vi "main.vi"() -> ()   [LabVIEW 2023] (continued)
2E\t80\tFF\tFF\tFD\r\n      1763  0CF101A7   00000004    8        68\t00\t97\tCC\t00\t16\t39\t72\r\n      1762  1FFFFFFF   00000004    8        00\t00\tFF\tFF\tFF\tFF\tFF\tFF\r\n      1803  0CF102A7   00000004    8        30\t75\tE0\t2E\t80\tFF\tFF\tFD\r\n      1803  0CF101A7   00000004    8        68\t00\t97\tCC\t00\t16\t39\t74\r\n      1802  1FFFFFFF   00000004    8        00\t00\tFF\tFF\tFF\tFF\tFF\tFF\r\n      1793  18F106A7   00000004    8        00\tF7\tFF\tFF\tFF\tFF\tFF\t94\r\n      1792  1FFFFFFF   00000004    8        00\t20\tFF\tFF\tFF\tFF\tFF\tFF\r\n      1783  0CF102A7   00000004    8        30\t75\tE0\t2E\t80\tFF\tFF\tFD\r\n      1783  0CF101A7   00000004    8        68\t00\t97\tCC\t00\t16\t39\t73\r\n      1782  1FFFFFFF   00000004    8        00\t20\tFF\tFF\tFF\tFF\tFF\tFF\r\n      1772  1FFFFFFF   00000004    8        00\t20\tFF\tFF\tFF\tFF\tFF\tFF\r\n      1763  0CF102A7   00000004    8        30\t75\tE0\t2E\t80\tFF\tFF\tFD\r\n      1763  0CF101A7   00000004    8        68\t00\t97\tCC\t00\t16\t39\t72\r\n      1812  1FFFFFFF   00000004    8        00\t20\tFF\tFF\tFF\tFF\tFF\tFF\r\n      1803  0CF102A7   00000004    8        30\t75\tE0\t2E\t80\tFF\tFF\tFD\r\n      1803  0CF101A7   00000004    8        68\t00\t97\tCC\t00\t16\t39\t74\r\n      1802  1FFFFFFF   00000004    8        00\t00\tFF\tFF\tFF\tFF\tFF\tFF\r\n      1793  18F106A7   00000004    8        00\tF7\tFF\tFF\tFF\tFF\tFF\t94\r\n      1792  1FFFFFFF   00000004    8        00\t20\tFF\tFF\tFF\tFF\tFF\tFF\r\n      1783  0CF102A7   00000004    8        30\t75\tE0\t2E\t80\tFF\tFF\tFD\r\n      1783  0CF101A7   00000004    8        68\t00\t97\tCC\t00\t16\t39\t73\r\n      1782  1FFFFFFF   00000004    8        00\t20\tFF\tFF\tFF\tFF\tFF\tFF\r\n      1772  1FFFFFFF   00000004    8        00\t20\tFF\tFF\tFF\tFF\tFF\tFF\r\n      1763  0CF102A7   00000004    8        30\t75\tE0\t2E\t80\tFF\tFF\tFD\r\n      1822  1FFFFFFF   00000004    8        00\t00\tFF\tFF\tFF\tFF\tFF\tFF\r\n      1812  1FFFFFFF   00000004    8        00\t20\tFF\tFF\tFF\tFF\tFF\tFF\r\n      1803  0CF102A7   00000004    8        30\t75\tE0\t2E\t80\tFF\tFF\tFD\r\n      1803  0CF101A7   00000004    8        68\t00\t97\tCC\t00\t16\t39\t74\r\n      1802  1FFFFFFF   00000004    8        00\t00\tFF\tFF\tFF\tFF\tFF\tFF\r\n      1793  18F106A7   00000004    8        00\tF7\tFF\tFF\tFF\tFF\tFF\t94\r\n      1792  1FFFFFFF   00000004    8        00\t20\tFF\tFF\tFF\tFF\tFF\tFF\r\n      1783  0CF102A7   00000004    8        30\t75\tE0\t2E\t80\tFF\tFF\tFD\r\n      1783  0CF101A7   00000004    8        68\t00\t97\tCC\t00\t16\t39\t73\r\n      1782  1FFFFFFF   00000004    8        00\t20\tFF\tFF\tFF\tFF\tFF\tFF\r\n      1772  1FFFFFFF   00000004    8        00\t20\tFF\tFF\tFF\tFF\tFF\tFF\r\n      1823  0CF101A7   00000004    8        68\t00\t97\tCC\t00\t16\t39\t75\r\n      1822  1FFFFFFF   00000004    8        00\t00\tFF\tFF\tFF\tFF\tFF\tFF\r\n      1812  1FFFFFFF   00000004    8        00\t20\tFF\tFF\tFF\tFF\tFF\tFF\r\n      1803  0CF102A7   00000004    8        30\t75\tE0\t2E\t80\tFF\tFF\tFD\r\n      1803  0CF101A7   00000004    8        68\t00\t97\tCC\t00\t16\t39\t74\r\n      1802  1FFFFFFF   00000004    8        00\t00\tFF\tFF\tFF\tFF\tFF\tFF\r\n      1793  18F106A7   00000004    8        00\tF7\tFF\tFF\tFF\tFF\tFF\t94\r\n      1792  1FFFFFFF   00000004    8        00\t20\tFF\tFF\tFF\tFF\tFF\tFF\r\n      1783  0CF102A7   00000004    8        30\t75\tE0\t2E\t80\tFF\tFF\tFD\r\n      1783  0CF101A7   00000004    8        68\t00\t97\tCC\t00\t16\t39\t73\r\n      1782  1FFFFFFF   00000004    8        00\t20\tFF\tFF\tFF\tFF\tFF\tFF\r\n      1823  0CF102A7   00000004    8        30\t75\tE0\t2E\t80\tFF\tFF\tFD\r\n      1823  0CF101A7   00000004    8        68\t00\t97\tCC\t00\t16\t39\t75\r\n      1822  1FFFFFFF   00000004    8        00\t00\tFF\tFF\tFF\tFF\tFF\tFF\r\n      1812  1FFFFFFF   00000004    8        00\t20\tFF\tFF\tFF\tFF\tFF\tFF\r\n      1803  0CF102A7   00000004    8        30\t75\tE0\t2E\t80\tFF\tFF\tFD\r\n      1803  0CF101A7   00000004    8        68\t00\t97\tCC\t00\t16\t39\t74\r\n      1802  1FFFFFFF   00000004    8        00\t00\tFF\tFF\tFF\tFF\tFF\tFF\r\n      1793  18F106A7   00000004    8        00\tF7\tFF\tFF\tFF\tFF\tFF\t94\r\n      1792  1FFFFFFF   00000004    8        00\t20\tFF\tFF\tFF\tFF\tFF\tFF\r\n      1783  0CF102A7   00000004    8        30\t75\tE0\t2E\t80\tFF\tFF\tFD\r\n      1783  0CF101A7   00000004    8        68\t00\t97\tCC\t00\t16\t39\t73\r\n      1832  1FFFFFFF   00000004    8        00\t20\tFF\tFF\tFF\tFF\tFF\tFF\r\n      1823  0CF102A7   00000004    8        30\t75\tE0\t2E\t80\tFF\tFF\tFD\r\n      1823  0CF101A7   00000004    8        68\t00\t97\tCC\t00\t16\t39\t75\r\n      1822  1FFFFFFF   00000004    8        00\t00\tFF\tFF\tFF\tFF\tFF\tFF\r\n      1812  1FFFFFFF   00000004    8        00\t20\tFF\tFF\tFF\tFF\tFF\tFF\r\n      1803  0CF102A7   00000004    8        30\t75\tE0\t2E\t80\tFF\tFF\tFD\r\n      1803  0CF101A7   00000004    8        68\t00\t97\tCC\t00\t16\t39\t74\r\n      1802  1FFFFFFF   00000004    8        00\t00\tFF\tFF\tFF\tFF\tFF\tFF\r\n      1793  18F106A7   00000004    8        00\tF7\tFF\tFF\tFF\tFF\tFF\t94\r\n      1792  1FFFFFFF   00000004    8        00\t20\tFF\tFF\tFF\tFF\tFF\tFF\r\n      1783  0CF102A7   00000004    8        30\t75\tE0\t2E\t80\tFF\tFF\tFD\r\n      1841  18F11FF0   00000004    8        FF\t3F\t90\t68\t88\t1B\t10\tAC\r\n      1832  1FFFFFFF   00000004    8        00\t20\tFF\tFF\tFF\tFF\tFF\tFF\r\n      1823  0CF102A7   00000004    8        30\t75\tE0\t2E\t80\tFF\tFF\tFD\r\n      1823  0CF101A7   00000004    8        68\t00\t97\tCC\t00\t16\t39\t75\r\n      1822  1FFFFFFF   00000004    8        00\t00\tFF\tFF\tFF\tFF\tFF\tFF\r\n      1812  1FFFFFFF   00000004    8        00\t20\tFF\tFF\tFF\tFF\tFF\tFF\r\n      1803  0CF102A7   00000004    8        30\t75\tE0\t2E\t80\tFF\tFF\tFD\r\n      1803  0CF101A7   00000004    8        68\t00\t97\tCC\t00\t16\t39\t74\r\n      1802  1FFFFFFF   00000004    8        00\t00\tFF\tFF\tFF\tFF\tFF\tFF\r\n      1793  18F106A7   00000004    8        00\tF7\tFF\tFF\tFF\tFF\tFF\t94\r\n      1792  1FFFFFFF   00000004    8        00\t20\tFF\tFF\tFF\tFF\tFF\tFF\r\n      1842  18F120F0   00000004    8        2B\t75\t60\tB1\tB0\t01\tFF\tFF\r\n      1841  18F11FF0   00000004    8        FF\t3F\t90\t68\t88\t1B\t10\tAC\r\n      1832  1FFFFFFF   00000004    8        00\t20\tFF\tFF\tFF\tFF\tFF\tFF\r\n      1823  0CF102A7   00000004    8        30\t75\tE0\t2E\t80\tFF\tFF\tFD\r\n      1823  0CF101A7   00000004    8        68\t00\t97\tCC\t00\t16\t39\t75\r\n      1822  1FFFFFFF   00000004    8        00\t00\tFF\tFF\tFF\tFF\tFF\tFF\r\n      1812  1FFFFFFF   00000004    8        00\t20\tFF\tFF\tFF\tFF\tFF\tFF\r\n      1803  0CF102A7   00000004    8        30\t75\tE0\t2E\t80\tFF\tFF\tFD\r\n      1803  0CF101A7   00000004    8        68\t00\t97\tCC\t00\t16\t39\t74\r\n      1802  1FFFFFFF   00000004    8        00\t00\tFF\tFF\tFF\tFF\tFF\tFF\r\n      1793  18F106A7   00000004    8        00\tF7\tFF\tFF\tFF\tFF\tFF\t94\r\n      1843  0CF101A7   00000004    8        68\t00\t97\tCC\t00\t16\t39\t76\r\n      1842  18F120F0   00000004    8        2B\t75\t60\tB1\tB0\t01\tFF\tFF\r\n      1841  18F11FF0   00000004    8        FF\t3F\t90\t68\t88\t1B\t10\tAC\r\n      1832  1FFFFFFF   00000004    8        00\t20\tFF\tFF\tFF\tFF\tFF\tFF\r\n      1823  0CF102A7   00000004    8        30\t75\tE0\t2E\t80\tFF\tFF\tFD\r\n      1823  0CF101A7   00000004    8        68\t00\t97\tCC\t00\t16\t39\t75\r\n      1822  1FFFFFFF   00000004    8        00\t00\tFF\tFF\tFF\tFF\tFF\tFF\r\n      1812  1FFFFFFF   00000004    8        00\t20\tFF\tFF\tFF\tFF\tFF\tFF\r\n      1803  0CF102A7   00000004    8        30\t75\tE0\t2E\t80\tFF\tFF\tFD\r\n      1803  0CF101A7   00000004    8        68\t00\t97\tCC\t00\t16\t39\t74\r\n      1802  1FFFFFFF   00000004    8        00\t00\tFF\tFF\tFF\tFF\tFF\tFF\r\n      1843  0C3C4D4A   00000004    8        BE\tFF\tFF\t7F\t18\tFF\tFF\t4A\r\n      1843  0CF101A7   00000004    8        68\t00\t97\tCC\t00\t16\t39\t76\r\n      1842  18F120F0   00000004    8        2B\t75\t60\tB1\tB0\t01\tFF\tFF\r\n      1841  18F11FF0   00000004    8        FF\t3F\t90\t68\t88\t1B\t10\tAC\r\n      1832  1FFFFFFF   00000004    8        00\t20\tFF\tFF\tFF\tFF\tFF\tFF\r\n      1823  0CF102A7   00000004    8        30\t75\tE0\t2E\t80\tFF\tFF\tFD\r\n      1823  0CF101A7   00000004    8        68\t00\t97\tCC\t00\t16\t39\t75\r\n      1822  1FFFFFFF   00000004    8        00\t00\tFF\tFF\tFF\tFF\tFF\tFF\r\n      1812  1FFFFFFF   00000004    8        00\t20\tFF\tFF\tFF\tFF\tFF\tFF\r\n      1803  0CF102A7   00000004    8        30\t75\tE0\t2E\t80\tFF\tFF\tFD\r\n      1803  0CF101A7   00000004    8        68\t00\t97\tCC\t00\t16\t39\t74\r\n      1844  0CF102A7   00000004    8        30\t75\tE0\t2E\t80\tFF\tFF\tFD\r\n      1843  0C3C4D4A   00000004    8        BE\tFF\tFF\t7F\t18\tFF\tFF\t4A\r\n      1843  0CF101A7   00000004    8        68\t00\t97\tCC\t00\t16\t39\t76\r\n      1842  18F120F0   00000004    8        2B\t75\t60\tB1\tB0\t01\tFF\tFF\r\n      1841  18F11FF0   00000004    8        FF\t3F\t90\t68\t88\t1B\t10\tAC\r\n      1832  1FFFFFFF   00000004    8        00\t20\tFF\tFF\tFF\tFF\tFF\tFF\r\n      1823  0CF102A7   00000004    8        30\t75\tE0\t2E\t80\tFF\tFF\tFD\r\n      1823  0CF101A7   00000004    8        68\t00\t97\tCC\t00\t16\t39\t75\r\n      1822  1FFFFFFF   00000004    8        00\t00\tFF\tFF\tFF\tFF\tFF\tFF\r\n      1812  1FFFFFFF   00000004    8        00\t20\tFF\tFF\tFF\tFF\tFF\tFF\r\n      1803  0CF102A7   00000004    8        30\t75\tE0\t2E\t80\tFF\tFF\tFD\r\n      1844  0CF103A7   00000004    8        17\t1F\t08\t60\tB1\t1F\t08\t4A\r\n      1844  0CF102A7   00000004    8        30\t75\tE0\t2E\t80\tFF\tFF\tFD\r\n      1843  0C3C4D4A   00000004    8        BE\tFF\tFF\t7F\t18\tFF\tFF\t4A\r\n      1843  0CF101A7   00000004    8        68\t00\t97\tCC\t00\t16\t39\t76\r\n      1842  18F120F0   00000004    8        2B\t75\t60\tB1\tB0\t01\tFF\tFF\r\n      1841  18F11FF0   00000004    8        FF\t3F\t90\t68\t88\t1B\t10\tAC\r\n      1832  1FFFFFFF   00000004    8        00\t20\tFF\tFF\tFF\tFF\tFF\tFF\r\n      1823  0CF102A7   00000004    8        30\t75\tE0\t2E\t80\tFF\tFF\tFD\r\n      1823  0CF101A7   00000004    8        68\t00\t97\tCC\t00\t16\t39\t75\r\n      1822  1FFFFFFF   00000004    8        00\t00\tFF\tFF\tFF\tFF\tFF\tFF\r\n      1812  1FFFFFFF   00000004    8        00\t20\tFF\tFF\tFF\tFF\tFF\tFF\r\n      1845  0CF104A7   00000004    8        F0\t60\t22\tFC\tFF\tFF\tFF\t4A\r\n      1844  0CF103A7   00000004    8        17\t1F\t08\t60\tB1\t1F\t08\t4A\r\n      1844  0CF102A7   00000004    8        30\t75\tE0\t2E\t80\tFF\tFF\tFD\r\n      1843  0C3C4D4A   00000004    8        BE\tFF\tFF\t7F\t18\tFF\tFF\t4A\r\n      1843  0CF101A7   00000004    8        68\t00\t97\tCC\t00\t16\t39\t76\r\n      1842  18F120F0   00000004    8        2B\t75\t60\tB1\tB0\t01\tFF\tFF\r\n      1841  18F11FF0   00000004    8        FF\t3F\t90\t68\t88\t1B\t10\tAC\r\n      1832  1FFFFFFF   00000004    8        00\t20\tFF\tFF\tFF\tFF\tFF\tFF\r\n      1823  0CF102A7   00000004    8        30\t75\tE0\t2E\t80\tFF\tFF\tFD\r\n      1823  0CF101A7   00000004    8        68\t00\t97\tCC\t00\t16\t39\t75\r\n      1822  1FFFFFFF   00000004    8        00\t00\tFF\tFF\tFF\tFF\tFF\tFF\r\n      1845  18F106A7   00000004    8        00\tF7\tFF\tFF\tFF\tFF\tFF\t95\r\n      1845  0CF104A7   00000004    8        F0\t60\t22\tFC\tFF\tFF\tFF\t4A\r\n      1844  0CF103A7   00000004    8        17\t1F\t08\t60\tB1\t1F\t08\t4A\r\n      1844  0CF102A7   00000004    8        30\t75\tE0\t2E\t80\tFF\tFF\tFD\r\n      1843  0C3C4D4A   00000004    8        BE\tFF\tFF\t7F\t18\tFF\tFF\t4A\r\n      1843  0CF101A7   00000004    8        68\t00\t97\tCC\t00\t16\t39\t76\r\n      1842  18F120F0   00000004    8        2B\t75\t60\tB1\tB0\t01\tFF\tFF\r\n      1841  18F11FF0   00000004    8        FF\t3F\t90\t68\t88\t1B\t10\tAC\r\n      1832  1FFFFFFF   00000004    8        00\t20\tFF\tFF\tFF\tFF\tFF\tFF\r\n      1823  0CF102A7   00000004    8        30\t75\tE0\t2E\t80\tFF\tFF\tFD\r\n      1823  0CF101A7   00000004    8        68\t00\t97\tCC\t00\t16\t39\t75\r\n      1846  18F121F0   00000004    8        09\t18\t00\t00\tFF\tFF\tB0\t01\r\n      1845  18F106A7   00000004    8        00\tF7\tFF\tFF\tFF\tFF\tFF\t95\r\n      1845  0CF104A7   00000004    8        F0\t60\t22\tFC\tFF\tFF\tFF\t4A\r\n      1844  0CF103A7   00000004    8        17\t1F\t08\t60\tB1\t1F\t08\t4A\r\n      1844  0CF102A7   00000004    8        30\t75\tE0\t2E\t80\tFF\tFF\tFD\r\n      1843  0C3C4D4A   00000004    8        BE\tFF\tFF\t7F\t18\tFF\tFF\t4A\r\n      1843  0CF101A7   00000004    8        68\t00\t97\tCC\t00\t16\t39\t76\r\n      1842  18F120F0   00000004    8        2B\t75\t60\tB1\tB0\t01\tFF\tFF\r\n      1841  18F11FF0   00000004    8        FF\t3F\t90\t68\t88\t1B\t10\tAC\r\n      1832  1FFFFFFF   00000004    8        00\t20\tFF\tFF\tFF\tFF\tFF\tFF\r\n      1823  0CF102A7   00000004    8        30\t75\tE0\t2E\t80\tFF\tFF\tFD\r\n      1847  1FFFFFFF   00000004    8        00\t00\tFF\tFF\tFF\tFF\tFF\tFF\r\n      1846  18F121F0   00000004    8        09\t18\t00\t00\tFF\tFF\tB0\t01\r\n      1845  18F106A7   00000004    8        00\tF7\tFF\tFF\tFF\tFF\tFF\t95\r\n      1845  0CF104A7   00000004    8        F0\t60\t22\tFC\tFF\tFF\tFF\t4A\r\n      1844  0CF103A7   00000004    8        17\t1F\t08\t60\tB1\t1F\t08\t4A\r\n      1844  0CF102A7   00000004    8        30\t75\tE0\t2E\t80\tFF\tFF\tFD\r\n      1843  0C3C4D4A   00000004    8        BE\tFF\tFF\t7F\t18\tFF\tFF\t4A\r\n      1843  0CF101A7   00000004    8        68\t00\t97\tCC\t00\t16\t39\t76\r\n      1842  18F120F0   00000004    8        2B\t75\t60\tB1\tB0\t01\tFF\tFF\r\n      1841  18F11FF0   00000004    8        FF\t3F\t90\t68\t88\t1B\t10\tAC\r\n      1832  1FFFFFFF   00000004    8        00\t20\tFF\tFF\tFF\tFF\tFF\tFF\r\n      1852  1FFFFFFF   00000004    8        00\t20\tFF\tFF\tFF\tFF\tFF\tFF\r\n      1847  1FFFFFFF   00000004    8        00\t00\tFF\tFF\tFF\tFF\tFF\tFF\r\n      1846  18F121F0   00000004    8        09\t18\t00\t00\tFF\tFF\tB0\t01\r\n      1845  18F106A7   00000004    8        00\tF7\tFF\tFF\tFF\tFF\tFF\t95\r\n      1845  0CF104A7   00000004    8        F0\t60\t22\tFC\tFF\tFF\tFF\t4A\r\n      1844  0CF103A7   00000004    8        17\t1F\t08\t60\tB1\t1F\t08\t4A\r\n      1844  0CF102A7   00000004    8        30\t75\tE0\t2E\t80\tFF\tFF\tFD\r\n      1843  0C3C4D4A   00000004    8        BE\tFF\tFF\t7F\t18\tFF\tFF\t4A\r\n      1843  0CF101A7   00000004    8        68\t00\t97\tCC\t00\t16\t39\t76\r\n      1842  18F120F0   00000004    8        2B\t75\t60\tB1\tB0\t01\tFF\tFF\r\n      1841  18F11FF0   00000004    8        FF\t3F\t90\t68\t88\t1B\t10\tAC\r\n      1862  1FFFFFFF   00000004    8        00\t20\tFF\tFF\tFF\tFF\tFF\tFF\r\n      1852  1FFFFFFF   00000004    8        00\t20\tFF\tFF\tFF\tFF\tFF\tFF\r\n      1847  1FFFFFFF   00000004    8        00\t00\tFF\tFF\tFF\tFF\tFF\tFF\r\n      1846  18F121F0   00000004    8        09\t18\t00\t00\tFF\tFF\tB0\t01\r\n      1845  18F106A7   00000004    8        00\tF7\tFF\tFF\tFF\tFF\tFF\t95\r\n      1845  0CF104A7   00000004    8        F0\t60\t22\tFC\tFF\tFF\tFF\t4A\r\n      1844  0CF103A7   00000004    8        17\t1F\t08\t60\tB1\t1F\t08\t4A\r\n      1844  0CF102A7   00000004    8        30\t75\tE0\t2E\t80\tFF\tFF\tFD\r\n      1843  0C3C4D4A   00000004    8        BE\tFF\tFF\t7F\t18\tFF\tFF\t4A\r\n      1843  0CF101A7   00000004    8        68\t00\t97\tCC\t00\t16\t39\t76\r\n      1842  18F120F0   00000004    8        2B\t75\t60\tB1\tB0\t01\tFF\tFF\r\n      1863  0CF101A7   00000004    8        68\t00\t97\tCC\t00\t16\t39\t77\r\n      1862  1FFFFFFF   00000004    8        00\t20\tFF\tFF\tFF\tFF\tFF\tFF\r\n      1852  1FFFFFFF   00000004    8        00\t20\tFF\tFF\tFF\tFF\tFF\tFF\r\n      1847  1FFFFFFF   00000004    8        00\t00\tFF\tFF\tFF\tFF\tFF\tFF\r\n      1846  18F121F0   00000004    8        09\t18\t00\t00\tFF\tFF\tB0\t01\r\n      1845  18F106A7   00000004    8        00\tF7\tFF\tFF\tFF\tFF\tFF\t95\r\n      1845  0CF104A7   00000004    8        F0\t60\t22\tFC\tFF\tFF\tFF\t4A\r\n      1844  0CF103A7   00000004    8        17\t1F\t08\t60\tB1\t1F\t08\t4A\r\n      1844  0CF102A7   00000004    8        30\t75\tE0\t2E\t80\tFF\tFF\tFD\r\n      1843  0C3C4D4A   00000004    8        BE\tFF\tFF\t7F\t18\tFF\tFF\t4A\r\n      1843  0CF101A7   00000004    8        68\t00\t97\tCC\t00\t16\t39\t76\r\n      1863  0CF102A7   00000004    8        30\t75\tE0\t2E\t80\tFF\tFF\tFD\r\n      1863  0CF101A7   00000004    8        68\t00\t97\tCC\t00\t16\t39\t77\r\n      1862  1FFFFFFF   00000004    8        00\t20\tFF\tFF\tFF\tFF\tFF\tFF\r\n      1852  1FFFFFFF   00000004    8        00\t20\tFF\tFF\tFF\tFF\tFF\tFF\r\n      1847  1FFFFFFF   00000004    8        00\t00\tFF\tFF\tFF\tFF\tFF\tFF\r\n      1846  18F121F0   00000004    8        09\t18\t00\t00\tFF\tFF\tB0\t01\r\n      1845  18F106A7   00000004    8        00\tF7\tFF\tFF\tFF\tFF\tFF\t95\r\n      1845  0CF104A7   00000004    8        F0\t60\t22\tFC\tFF\tFF\tFF\t4A\r\n      1844  0CF103A7   00000004    8        17\t1F\t08\t60\tB1\t1F\t08\t4A\r\n      1844  0CF102A7   00000004    8        30\t75\tE0\t2E\t80\tFF\tFF\tFD\r\n      1843  0C3C4D4A   00000004    8        BE\tFF\tFF\t7F\t18\tFF\tFF\t4A\r\n      1872  1FFFFFFF   00000004    8        00\t20\tFF\tFF\tFF\tFF\tFF\tFF\r\n      1863  0CF102A7   00000004    8        30\t75\tE0\t2E\t80\tFF\tFF\tFD\r\n      1863  0CF101A7   00000004    8        68\t00\t97\tCC\t00\t16\t39\t77\r\n      1862  1FFFFFFF   00000004    8        00\t20\tFF\tFF\tFF\tFF\tFF\tFF\r\n      1852  1FFFFFFF   00000004    8        00\t20\tFF\tFF\tFF\tFF\tFF\tFF\r\n      1847  1FFFFFFF   00000004    8        00\t00\tFF\tFF\tFF\tFF\tFF\tFF\r\n      1846  18F121F0   00000004    8        09\t18\t00\t00\tFF\tFF\tB0\t01\r\n      1845  18F106A7   00000004    8        00\tF7\tFF\tFF\tFF\tFF\tFF\t95\r\n      1845  0CF104A7   00000004    8        F0\t60\t22\tFC\tFF\tFF\tFF\t4A\r\n      1844  0CF103A7   00000004    8        17\t1F\t08\t60\tB1\t1F\t08\t4A\r\n      1844  0CF102A7   00000004    8        30\t75\tE0\t2E\t80\tFF\tFF\tFD\r\n      1882  1FFFFFFF   00000004    8        00\t20\tFF\tFF\tFF\tFF\tFF\tFF\r\n      1872  1FFFFFFF   00000004    8        00\t20\tFF\tFF\tFF\tFF\tFF\tFF\r\n      1863  0CF102A7   00000004    8        30\t75\tE0\t2E\t80\tFF\tFF\tFD\r\n      1863  0CF101A7   00000004    8        68\t00\t97\tCC\t00\t16\t39\t77\r\n      1862  1FFFFFFF   00000004    8        00\t20\tFF\tFF\tFF\tFF\tFF\tFF\r\n      1852  1FFFFFFF   00000004    8        00\t20\tFF\tFF\tFF\tFF\tFF\tFF\r\n      1847  1FFFFFFF   00000004    8        00\t00\tFF\tFF\tFF\tFF\tFF\tFF\r\n      1846  18F121F0   00000004    8        09\t18\t00\t00\tFF\tFF\tB0\t01\r\n      1845  18F106A7   00000004    8        00\tF7\tFF\tFF\tFF\tFF\tFF\t95\r\n      1845  0CF104A7   00000004    8        F0\t60\t22\tFC\tFF\tFF\tFF\t4A\r\n      1844  0CF103A7   00000004    8        17\t1F\t08\t60\tB1\t1F\t08\t4A\r\n      1883  0CF101A7   00000004    8        68\t00\t97\tCC\t00\t16\t39\t78\r\n      1882  1FFFFFFF   00000004    8        00\t20\tFF\tFF\tFF\tFF\tFF\tFF\r\n      1872  1FFFFFFF   00000004    8        00\t20\tFF\tFF\tFF\tFF\tFF\tFF\r\n      1863  0CF102A7   00000004    8        30\t75\tE0\t2E\t80\tFF\tFF\tFD\r\n      1863  0CF101A7   00000004    8        68\t00\t97\tCC\t00\t16\t39\t77\r\n      1862  1FFFFFFF   00000004    8        00\t20\tFF\tFF\tFF\tFF\tFF\tFF\r\n      1852  1FFFFFFF   00000004    8        00\t20\tFF\tFF\tFF\tFF\tFF\tFF\r\n      1847  1FFFFFFF   00000004    8        00\t00\tFF\tFF\tFF\tFF\tFF\tFF\r\n      1846  18F121F0   00000004    8        09\t18\t00\t00\tFF\tFF\tB0\t01\r\n      1845  18F106A7   00000004    8        00\tF7\tFF\tFF\tFF\tFF\tFF\t95\r\n      1845  0CF104A7   00000004    8        F0\t60\t22\tFC\tFF\tFF\tFF\t4A\r\n      1883  0CF102A7   00000004    8        30\t75\tE0\t2E\t80\tFF\tFF\tFD\r\n      1883  0CF101A7   00000004    8        68\t00\t97\tCC\t00\t16\t39\t78\r\n      1882  1FFFFFFF   00000004    8        00\t20\tFF\tFF\tFF\tFF\tFF\tFF\r\n      1872  1FFFFFFF   00000004    8        00\t20\tFF\tFF\tFF\tFF\tFF\tFF\r\n      1863  0CF102A7   00000004    8        30\t75\tE0\t2E\t80\tFF\tFF\tFD\r\n      1863  0CF101A7   00000004    8        68\t00\t97\tCC\t00\t16\t39\t77\r\n      1862  1FFFFFFF   00000004    8        00\t20\tFF\tFF\tFF\tFF\tFF\tFF\r\n      1852  1FFFFFFF   00000004    8        00\t20\tFF\tFF\tFF\tFF\tFF\tFF\r\n      1847  1FFFFFFF   00000004    8        00\t00\tFF\tFF\tFF\tFF\tFF\tFF\r\n      1846  18F121F0   00000004    8        09\t18\t00\t00\tFF\tFF\tB0\t01\r\n      1845  18F106A7   00000004    8        00\tF7\tFF\tFF\tFF\tFF\tFF\t95\r\n      1892  1FFFFFFF   00000004    8        00\t00\tFF\tFF\tFF\tFF\tFF\tFF\r\n      1883  0CF102A7   00000004    8        30\t75\tE0\t2E\t80\tFF\tFF\tFD\r\n      1883  0CF101A7   00000004    8        68\t00\t97\tCC\t00\t16\t39\t78\r\n      1882  1FFFFFFF   00000004    8        00\t20\tFF\tFF\tFF\tFF\tFF\tFF\r\n      1872  1FFFFFFF   00000004    8        00\t20\tFF\tFF\tFF\tFF\tFF\tFF\r\n      1863  0CF102A7   00000004    8        30\t75\tE0\t2E\t80\tFF\tFF\tFD\r\n      1863  0CF101A7   00000004    8        68\t00\t97\tCC\t00\t16\t39\t77\r\n      1862  1FFFFFFF   00000004    8        00\t20\tFF\tFF\tFF\tFF\tFF\tFF\r\n      1852  1FFFFFFF   00000004    8        00\t20\tFF\tFF\tFF\tFF\tFF\tFF\r\n      1847  1FFFFFFF   00000004    8        00\t00\tFF\tFF\tFF\tFF\tFF\tFF\r\n      1846  18F121F0   00000004    8        09\t18\t00\t00\tFF\tFF\tB0\t01\r\n      1893  18F106A7   00000004    8        00\tF7\tFF\tFF\tFF\tFF\tFF\t96\r\n      1892  1FFFFFFF   00000004    8        00\t00\tFF\tFF\tFF\tFF\tFF\tFF\r\n      1883  0CF102A7   00000004    8        30\t75\tE0\t2E\t80\tFF\tFF\tFD\r\n      1883  0CF101A7   00000004    8        68\t00\t97\tCC\t00\t16\t39\t78\r\n      1882  1FFFFFFF   00000004    8        00\t20\tFF\tFF\tFF\tFF\tFF\tFF\r\n      1872  1FFFFFFF   00000004    8        00\t20\tFF\tFF\tFF\tFF\tFF\tFF\r\n      1863  0CF102A7   00000004    8        30\t75\tE0\t2E\t80\tFF\tFF\tFD\r\n      1863  0CF101A7   00000004    8        68\t00\t97\tCC\t00\t16\t39\t77\r\n      1862  1FFFFFFF   00000004    8        00\t20\tFF\tFF\tFF\tFF\tFF\tFF\r\n      1852  1FFFFFFF   00000004    8        00\t20\tFF\tFF\tFF\tFF\tFF\tFF\r\n      1847  1FFFFFFF   00000004    8        00\t00\tFF\tFF\tFF\tFF\tFF\tFF\r\n      1902  1FFFFFFF   00000004    8        00\t20\tFF\tFF\tFF\tFF\tFF\tFF\r\n      1893  18F106A7   00000004    8        00\tF7\tFF\tFF\tFF\tFF\tFF\t96\r\n      1892  1FFFFFFF   00000004    8        00\t00\tFF\tFF\tFF\tFF\tFF\tFF\r\n      1883  0CF102A7   00000004    8        30\t75\tE0\t2E\t80\tFF\tFF\tFD\r\n      1883  0CF101A7   00000004    8        68\t00\t97\tCC\t00\t16\t39\t78\r\n      1882  1FFFFFFF   00000004    8        00\t20\tFF\tFF\tFF\tFF\tFF\tFF\r\n      1872  1FFFFFFF   00000004    8        00\t20\tFF\tFF\tFF\tFF\tFF\tFF\r\n      1863  0CF102A7   00000004    8        30\t75\tE0\t2E\t80\tFF\tFF\tFD\r\n      1863  0CF101A7   00000004    8        68\t00\t97\tCC\t00\t16\t39\t77\r\n      1862  1FFFFFFF   00000004    8        00\t20\tFF\tFF\tFF\tFF\tFF\tFF\r\n      1852  1FFFFFFF   00000004    8        00\t20\tFF\tFF\tFF\tFF\tFF\tFF\r\n      1903  0CF101A7   00000004    8        68\t00\t97\tCC\t00\t16\t39\t79\r\n      1902  1FFFFFFF   00000004    8        00\t20\tFF\tFF\tFF\tFF\tFF\tFF\r\n      1893  18F106A7   00000004    8        00\tF7\tFF\tFF\tFF\tFF\tFF\t96\r\n      1892  1FFFFFFF   00000004    8        00\t00\tFF\tFF\tFF\tFF\tFF\tFF\r\n      1883  0CF102A7   00000004    8        30\t75\tE0\t2E\t80\tFF\tFF\tFD\r\n      1883  0CF101A7   00000004    8        68\t00\t97\tCC\t00\t16\t39\t78\r\n      1882  1FFFFFFF   00000004    8        00\t20\tFF\tFF\tFF\tFF\tFF\tFF\r\n      1872  1FFFFFFF   00000004    8        00\t20\tFF\tFF\tFF\tFF\tFF\tFF\r\n      1863  0CF102A7   00000004    8        30\t75\tE0\t2E\t80\tFF\tFF\tFD\r\n      1863  0CF101A7   00000004    8        68\t00\t97\tCC\t00\t16\t39\t77\r\n      1862  1FFFFFFF   00000004    8        00\t20\tFF\tFF\tFF\tFF\tFF\tFF\r\n      1903  0CF102A7   00000004    8        30\t75\tE0\t2E\t80\tFF\tFF\tFD\r\n      1903  0CF101A7   00000004    8        68\t00\t97\tCC\t00\t16\t39\t79\r\n      1902  1FFFFFFF   00000004    8        00\t20\tFF\tFF\tFF\tFF\tFF\tFF\r\n      1893  18F106A7   00000004    8        00\tF7\tFF\tFF\tFF\tFF\tFF\t96\r\n      1892  1FFFFFFF   00000004    8        00\t00\tFF\tFF\tFF\tFF\tFF\tFF\r\n      1883  0CF102A7   00000004    8        30\t75\tE0\t2E\t80\tFF\tFF\tFD\r\n      1883  0CF101A7   00000004    8        68\t00\t97\tCC\t00\t16\t39\t78\r\n      1882  1FFFFFFF   00000004    8        00\t20\tFF\tFF\tFF\tFF\tFF\tFF\r\n      1872  1FFFFFFF   00000004    8        00\t20\tFF\tFF\tFF\tFF\tFF\tFF\r\n      1863  0CF102A7   00000004    8        30\t75\tE0\t2E\t80\tFF\tFF\tFD\r\n      1863  0CF101A7   00000004    8        68\t00\t97\tCC\t00\t16\t39\t77\r\n      1912  1FFFFFFF   00000004    8        00\t00\tFF\tFF\tFF\tFF\tFF\tFF\r\n      1903  0CF102A7   00000004    8        30\t75\tE0\t2E\t80\tFF\tFF\tFD\r\n      1903  0CF101A7   00000004    8        68\t00\t97\tCC\t00\t16\t39\t79\r\n      1902  1FFFFFFF   00000004    8        00\t20\tFF\tFF\tFF\tFF\tFF\tFF\r\n      1893  18F106A7   00000004    8        00\tF7\tFF\tFF\tFF\tFF\tFF\t96\r\n      1892  1FFFFFFF   00000004    8        00\t00\tFF\tFF\tFF\tFF\tFF\tFF\r\n      1883  0CF102A7   00000004    8        30\t75\tE0\t2E\t80\tFF\tFF\tFD\r\n      1883  0CF101A7   00000004    8        68\t00\t97\tCC\t00\t16\t39\t78\r\n      1882  1FFFFFFF   00000004    8        00\t20\tFF\tFF\tFF\tFF\tFF\tFF\r\n      1872  1FFFFFFF   00000004    8        00\t20\tFF\tFF\tFF\tFF\tFF\tFF\r\n      1863  0CF102A7   00000004    8        30\t75\tE0\t2E\t80\tFF\tFF\tFD\r\n      1922  1FFFFFFF   00000004    8        00\t20\tFF\tFF\tFF\tFF\tFF\tFF\r\n      1912  1FFFFFFF   00000004    8        00\t00\tFF\tFF\tFF\tFF\tFF\tFF\r\n      1903  0CF102A7   00000004    8        30\t75\tE0\t2E\t80\tFF\tFF\tFD\r\n      1903  0CF101A7   00000004    8        68\t00\t97\tCC\t00\t16\t39\t79\r\n      1902  1FFFFFFF   00000004    8        00\t20\tFF\tFF\tFF\tFF\tFF\tFF\r\n      1893  18F106A7   00000004    8        00\tF7\tFF\tFF\tFF\tFF\tFF\t96\r\n      1892  1FFFFFFF   00000004    8        00\t00\tFF\tFF\tFF\tFF\tFF\tFF\r\n      1883  0CF102A7   00000004    8        30\t75\tE0\t2E\t80\tFF\tFF\tFD\r\n      1883  0CF101A7   00000004    8        68\t00\t97\tCC\t00\t16\t39\t78\r\n      1882  1FFFFFFF   00000004    8        00\t20\tFF\tFF\tFF\tFF\tFF\tFF\r\n      1872  1FFFFFFF   00000004    8        00\t20\tFF\tFF\tFF\tFF\tFF\tFF\r\n      1923  0CF101A7   00000004    8        68\t00\t97\tCC\t00\t16\t39\t7A\r\n      1922  1FFFFFFF   00000004    8        00\t20\tFF\tFF\tFF\tFF\tFF\tFF\r\n      1912  1FFFFFFF   00000004    8        00\t00\tFF\tFF\tFF\tFF\tFF\tFF\r\n      1903  0CF102A7   00000004    8        30\t75\tE0\t2E\t80\tFF\tFF\tFD\r\n      1903  0CF101A7   00000004    8        68\t00\t97\tCC\t00\t16\t39\t79\r\n      1902  1FFFFFFF   00000004    8        00\t20\tFF\tFF\tFF\tFF\tFF\tFF\r\n      1893  18F106A7   00000004    8        00\tF7\tFF\tFF\tFF\tFF\tFF\t96\r\n      1892  1FFFFFFF   00000004    8        00\t00\tFF\tFF\tFF\tFF\tFF\tFF\r\n      1883  0CF102A7   00000004    8        30\t75\tE0\t2E\t80\tFF\tFF\tFD\r\n      1883  0CF101A7   00000004    8        68\t00\t97\tCC\t00\t16\t39\t78\r\n      1882  1FFFFFFF   00000004    8        00\t20\tFF\tFF\tFF\tFF\tFF\tFF\r\n      1923  0CF102A7   00000004    8        30\t75\tE0\t2E\t80\tFF\tFF\tFD\r\n      1923  0CF101A7   00000004    8        68\t00\t97\tCC\t00\t16\t39\t7A\r\n      1922  1FFFFFFF   00000004    8        00\t20\tFF\tFF\tFF\tFF\tFF\tFF\r\n      1912  1FFFFFFF   00000004    8        00\t00\tFF\tFF\tFF\tFF\tFF\tFF\r\n      1903  0CF102A7   00000004    8        30\t75\tE0\t2E\t80\tFF\tFF\tFD\r\n      1903  0CF101A7   00000004    8        68\t00\t97\tCC\t00\t16\t39\t79\r\n      1902  1FFFFFFF   00000004    8        00\t20\tFF\tFF\tFF\tFF\tFF\tFF\r\n      1893  18F106A7   00000004    8        00\tF7\tFF\tFF\tFF\tFF\tFF\t96\r\n      1892  1FFFFFFF   00000004    8        00\t00\tFF\tFF\tFF\tFF\tFF\tFF\r\n      1883  0CF102A7   00000004    8        30\t75\tE0\t2E\t80\tFF\tFF\tFD\r\n      1883  0CF101A7   00000004    8        68\t00\t97\tCC\t00\t16\t39\t78\r\n      1932  1FFFFFFF   00000004    8        00\t20\tFF\tFF\tFF\tFF\tFF\tFF\r\n      1923  0CF102A7   00000004    8        30\t75\tE0\t2E\t80\tFF\tFF\tFD\r\n      1923  0CF101A7   00000004    8        68\t00\t97\tCC\t00\t16\t39\t7A\r\n      1922  1FFFFFFF   00000004    8        00\t20\tFF\tFF\tFF\tFF\tFF\tFF\r\n      1912  1FFFFFFF   00000004    8        00\t00\tFF\tFF\tFF\tFF\tFF\tFF\r\n      1903  0CF102A7   00000004    8        30\t75\tE0\t2E\t80\tFF\tFF\tFD\r\n      1903  0CF101A7   00000004    8        68\t00\t97\tCC\t00\t16\t39\t79\r\n      1902  1FFFFFFF   00000004    8        00\t20\tFF\tFF\tFF\tFF\tFF\tFF\r\n      1893  18F106A7   00000004    8        00\tF7\tFF\tFF\tFF\tFF\tFF\t96\r\n      1892  1FFFFFFF   00000004    8        00\t00\tFF\tFF\tFF\tFF\tFF\tFF\r\n      1883  0CF102A7   00000004    8        30\t75\tE0\t2E\t80\tFF\tFF\tFD\r\n      1941  18F11FF0   00000004    8        FF\t3F\t90\t68\t88\t1B\t10\tBC\r\n      1932  1FFFFFFF   00000004    8        00\t20\tFF\tFF\tFF\tFF\tFF\tFF\r\n      1923  0CF102A7   00000004    8        30\t75\tE0\t2E\t80\tFF\tFF\tFD\r\n      1923  0CF101A7   00000004    8        68\t00\t97\tCC\t00\t16\t39\t7A\r\n      1922  1FFFFFFF   00000004    8        00\t20\tFF\tFF\tFF\tFF\tFF\tFF\r\n      1912  1FFFFFFF   00000004    8        00\t00\tFF\tFF\tFF\tFF\tFF\tFF\r\n      1903  0CF102A7   00000004    8        30\t75\tE0\t2E\t80\tFF\tFF\tFD\r\n      1903  0CF101A7   00000004    8        68\t00\t97\tCC\t00\t16\t39\t79\r\n      1902  1FFFFFFF   00000004    8        00\t20\tFF\tFF\tFF\tFF\tFF\tFF\r\n      1893  18F106A7   00000004    8        00\tF7\tFF\tFF\tFF\tFF\tFF\t96\r\n      1892  1FFFFFFF   00000004    8        00\t00\tFF\tFF\tFF\tFF\tFF\tFF\r\n      1942  18F120F0   00000004    8        2B\t75\t60\tB1\tB0\t01\tFF\tFF\r\n      1941  18F11FF0   00000004    8        FF\t3F\t90\t68\t88\t1B\t10\tBC\r\n      1932  1FFFFFFF   00000004    8        00\t20\tFF\tFF\tFF\tFF\tFF\tFF\r\n      1923  0CF102A7   00000004    8        30\t75\tE0\t2E\t80\tFF\tFF\tFD\r\n      1923  0CF101A7   00000004    8        68\t00\t97\tCC\t00\t16\t39\t7A\r\n      1922  1FFFFFFF   00000004    8        00\t20\tFF\tFF\tFF\tFF\tFF\tFF\r\n      1912  1FFFFFFF   00000004    8        00\t00\tFF\tFF\tFF\tFF\tFF\tFF\r\n      1903  0CF102A7   00000004    8        30\t75\tE0\t2E\t80\tFF\tFF\tFD\r\n      1903  0CF101A7   00000004    8        68\t00\t97\tCC\t00\t16\t39\t79\r\n      1902  1FFFFFFF   00000004    8        00\t20\tFF\tFF\tFF\tFF\tFF\tFF\r\n      1893  18F106A7   00000004    8        00\tF7\tFF\tFF\tFF\tFF\tFF\t96\r\n      1943  0CF101A7   00000004    8        68\t00\t97\tCC\t00\t16\t39\t7B\r\n      1942  18F120F0   00000004    8        2B\t75\t60\tB1\tB0\t01\tFF\tFF\r\n      1941  18F11FF0   00000004    8        FF\t3F\t90\t68\t88\t1B\t10\tBC\r\n      1932  1FFFFFFF   00000004    8        00\t20\tFF\tFF\tFF\tFF\tFF\tFF\r\n      1923  0CF102A7   00000004    8        30\t75\tE0\t2E\t80\tFF\tFF\tFD\r\n      1923  0CF101A7   00000004    8        68\t00\t97\tCC\t00\t16\t39\t7A\r\n      1922  1FFFFFFF   00000004    8        00\t20\tFF\tFF\tFF\tFF\tFF\tFF\r\n      1912  1FFFFFFF   00000004    8        00\t00\tFF\tFF\tFF\tFF\tFF\tFF\r\n      1903  0CF102A7   00000004    8        30\t75\tE0\t2E\t80\tFF\tFF\tFD\r\n      1903  0CF101A7   00000004    8        68\t00\t97\tCC\t00\t16\t39\t79\r\n      1902  1FFFFFFF   00000004    8        00\t20\tFF\tFF\tFF\tFF\tFF\tFF\r\n      1943  0C3C4D4A   00000004    8        BE\tFF\tFF\t7F\t18\tFF\tFF\t4B\r\n      1943  0CF101A7   00000004    8        68\t00\t97\tCC\t00\t16\t39\t7B\r\n      1942  18F120F0   00000004    8        2B\t75\t60\tB1\tB0\t01\tFF\tFF\r\n      1941  18F11FF0   00000004    8        FF\t3F\t90\t68\t88\t1B\t10\tBC\r\n      1932  1FFFFFFF   00000004    8        00\t20\tFF\tFF\tFF\tFF\tFF\tFF\r\n      1923  0CF102A7   00000004    8        30\t75\tE0\t2E\t80\tFF\tFF\tFD\r\n      1923  0CF101A7   00000004    8        68\t00\t97\tCC\t00\t16\t39\t7A\r\n      1922  1FFFFFFF   00000004    8        00\t20\tFF\tFF\tFF\tFF\tFF\tFF\r\n      1912  1FFFFFFF   00000004    8        00\t00\tFF\tFF\tFF\tFF\tFF\tFF\r\n      1903  0CF102A7   00000004    8        30\t75\tE0\t2E\t80\tFF\tFF\tFD\r\n      1903  0CF101A7   00000004    8        68\t00\t97\tCC\t00\t16\t39\t79\r\n      1944  0CF102A7   00000004    8        30\t75\tE0\t2E\t80\tFF\tFF\tFD\r\n      1943  0C3C4D4A   00000004    8        BE\tFF\tFF\t7F\t18\tFF\tFF\t4B\r\n      1943  0CF101A7   00000004    8        68\t00\t97\tCC\t00\t16\t39\t7B\r\n      1942  18F120F0   00000004    8        2B\t75\t60\tB1\tB0\t01\tFF\tFF\r\n      1941  18F11FF0   00000004    8        FF\t3F\t90\t68\t88\t1B\t10\tBC\r\n      1932  1FFFFFFF   00000004    8        00\t20\tFF\tFF\tFF\tFF\tFF\tFF\r\n      1923  0CF102A7   00000004    8        30\t75\tE0\t2E\t80\tFF\tFF\tFD\r\n      1923  0CF101A7   00000004    8        68\t00\t97\tCC\t00\t16\t39\t7A\r\n      1922  1FFFFFFF   00000004    8        00\t20\tFF\tFF\tFF\tFF\tFF\tFF\r\n      1912  1FFFFFFF   00000004    8        00\t00\tFF\tFF\tFF\tFF\tFF\tFF\r\n      1903  0CF102A7   00000004    8        30\t75\tE0\t2E\t80\tFF\tFF\tFD\r\n      1944  0CF103A7   00000004    8        17\t1F\t08\t60\tB1\t1F\t08\t4B\r\n      1944  0CF102A7   00000004    8        30\t75\tE0\t2E\t80\tFF\tFF\tFD\r\n      1943  0C3C4D4A   00000004    8        BE\tFF\tFF\t7F\t18\tFF\tFF\t4B\r\n      1943  0CF101A7   00000004    8        68\t00\t97\tCC\t00\t16\t39\t7B\r\n      1942  18F120F0   00000004    8        2B\t75\t60\tB1\tB0\t01\tFF\tFF\r\n      1941  18F11FF0   00000004    8        FF\t3F\t90\t68\t88\t1B\t10\tBC\r\n      1932  1FFFFFFF   00000004    8        00\t20\tFF\tFF\tFF\tFF\tFF\tFF\r\n      1923  0CF102A7   00000004    8        30\t75\tE0\t2E\t80\tFF\tFF\tFD\r\n      1923  0CF101A7   00000004    8        68\t00\t97\tCC\t00\t16\t39\t7A\r\n      1922  1FFFFFFF   00000004    8        00\t20\tFF\tFF\tFF\tFF\tFF\tFF\r\n      1912  1FFFFFFF   00000004    8        00\t00\tFF\tFF\tFF\tFF\tFF\tFF\r\n      1945  0CF104A7   00000004    8        F0\t60\t22\tFC\tFF\tFF\tFF\t4B\r\n      1944  0CF103A7   00000004    8        17\t1F\t08\t60\tB1\t1F\t08\t4B\r\n      1944  0CF102A7   00000004    8        30\t75\tE0\t2E\t80\tFF\tFF\tFD\r\n      1943  0C3C4D4A   00000004    8        BE\tFF\tFF\t7F\t18\tFF\tFF\t4B\r\n      1943  0CF101A7   00000004    8        68\t00\t97\tCC\t00\t16\t39\t7B\r\n      1942  18F120F0   00000004    8        2B\t75\t60\tB1\tB0\t01\tFF\tFF\r\n      1941  18F11FF0   00000004    8        FF\t3F\t90\t68\t88\t1B\t10\tBC\r\n      1932  1FFFFFFF   00000004    8        00\t20\tFF\tFF\tFF\tFF\tFF\tFF\r\n      1923  0CF102A7   00000004    8        30\t75\tE0\t2E\t80\tFF\tFF\tFD\r\n      1923  0CF101A7   00000004    8        68\t00\t97\tCC\t00\t16\t39\t7A\r\n      1922  1FFFFFFF   00000004    8        00\t20\tFF\tFF\tFF\tFF\tFF\tFF\r\n      1945  18F106A7   00000004    8        00\tF7\tFF\tFF\tFF\tFF\tFF\t97\r\n      1945  0CF104A7   00000004    8        F0\t60\t22\tFC\tFF\tFF\tFF\t4B\r\n      1944  0CF103A7   00000004    8        17\t1F\t08\t60\tB1\t1F\t08\t4B\r\n      1944  0CF102A7   00000004    8        30\t75\tE0\t2E\t80\tFF\tFF\tFD\r\n      1943  0C3C4D4A   00000004    8        BE\tFF\tFF\t7F\t18\tFF\tFF\t4B\r\n      1943  0CF101A7   00000004    8        68\t00\t97\tCC\t00\t16\t39\t7B\r\n      1942  18F120F0   00000004    8        2B\t75\t60\tB1\tB0\t01\tFF\tFF\r\n      1941  18F11FF0   00000004    8        FF\t3F\t90\t68\t88\t1B\t10\tBC\r\n      1932  1FFFFFFF   00000004    8        00\t20\tFF\tFF\tFF\tFF\tFF\tFF\r\n      1923  0CF102A7   00000004    8        30\t75\tE0\t2E\t80\tFF\tFF\tFD\r\n      1923  0CF101A7   00000004    8        68\t00\t97\tCC\t00\t16\t39\t7A\r\n      1946  18F121F0   00000004    8        09\t18\t00\t00\tFF\tFF\tB0\t01\r\n      1945  18F106A7   00000004    8        00\tF7\tFF\tFF\tFF\tFF\tFF\t97\r\n      1945  0CF104A7   00000004    8        F0\t60\t22\tFC\tFF\tFF\tFF\t4B\r\n      1944  0CF103A7   00000004    8        17\t1F\t08\t60\tB1\t1F\t08\t4B\r\n      1944  0CF102A7   00000004    8        30\t75\tE0\t2E\t80\tFF\tFF\tFD\r\n      1943  0C3C4D4A   00000004    8        BE\tFF\tFF\t7F\t18\tFF\tFF\t4B\r\n      1943  0CF101A7   00000004    8        68\t00\t97\tCC\t00\t16\t39\t7B\r\n      1942  18F120F0   00000004    8        2B\t75\t60\tB1\tB0\t01\tFF\tFF\r\n      1941  18F11FF0   00000004    8        FF\t3F\t90\t68\t88\t1B\t10\tBC\r\n      1932  1FFFFFFF   00000004    8        00\t20\tFF\tFF\tFF\tFF\tFF\tFF\r\n      1923  0CF102A7   00000004    8        30\t75\tE0\t2E\t80\tFF\tFF\tFD\r\n      1947  1FFFFFFF   00000004    8        00\t20\tFF\tFF\tFF\tFF\tFF\tFF\r\n      1946  18F121F0   00000004    8        09\t18\t00\t00\tFF\tFF\tB0\t01\r\n      1945  18F106A7   00000004    8        00\tF7\tFF\tFF\tFF\tFF\tFF\t97\r\n      1945  0CF104A7   00000004    8        F0\t60\t22\tFC\tFF\tFF\tFF\t4B\r\n      1944  0CF103A7   00000004    8        17\t1F\t08\t60\tB1\t1F\t08\t4B\r\n      1944  0CF102A7   00000004    8        30\t75\tE0\t2E\t80\tFF\tFF\tFD\r\n      1943  0C3C4D4A   00000004    8        BE\tFF\tFF\t7F\t18\tFF\tFF\t4B\r\n      1943  0CF101A7   00000004    8        68\t00\t97\tCC\t00\t16\t39\t7B\r\n      1942  18F120F0   00000004    8        2B\t75\t60\tB1\tB0\t01\tFF\tFF\r\n      1941  18F11FF0   00000004    8        FF\t3F\t90\t68\t88\t1B\t10\tBC\r\n      1932  1FFFFFFF   00000004    8        00\t20\tFF\tFF\tFF\tFF\tFF\tFF\r\n      1952  1FFFFFFF   00000004    8        00\t00\tFF\tFF\tFF\tFF\tFF\tFF\r\n      1947  1FFFFFFF   00000004    8        00\t20\tFF\tFF\tFF\tFF\tFF\tFF\r\n      1946  18F121F0   00000004    8        09\t18\t00\t00\tFF\tFF\tB0\t01\r\n      1945  18F106A7   00000004    8        00\tF7\tFF\tFF\tFF\tFF\tFF\t97\r\n      1945  0CF104A7   00000004    8        F0\t60\t22\tFC\tFF\tFF\tFF\t4B\r\n      1944  0CF103A7   00000004    8        17\t1F\t08\t60\tB1\t1F\t08\t4B\r\n      1944  0CF102A7   00000004    8        30\t75\tE0\t2E\t80\tFF\tFF\tFD\r\n      1943  0C3C4D4A   00000004    8        BE\tFF\tFF\t7F\t18\tFF\tFF\t4B\r\n      1943  0CF101A7   00000004    8        68\t00\t97\tCC\t00\t16\t39\t7B\r\n      1942  18F120F0   00000004    8        2B\t75\t60\tB1\tB0\t01\tFF\tFF\r\n      1941  18F11FF0   00000004    8        FF\t3F\t90\t68\t88\t1B\t10\tBC\r\n      1962  1FFFFFFF   00000004    8        00\t00\tFF\tFF\tFF\tFF\tFF\tFF\r\n      1952  1FFFFFFF   00000004    8        00\t00\tFF\tFF\tFF\tFF\tFF\tFF\r\n      1947  1FFFFFFF   00000004    8        00\t20\tFF\tFF\tFF\tFF\tFF\tFF\r\n      1946  18F121F0   00000004    8        09\t18\t00\t00\tFF\tFF\tB0\t01\r\n      1945  18F106A7   00000004    8        00\tF7\tFF\tFF\tFF\tFF\tFF\t97\r\n      1945  0CF104A7   00000004    8        F0\t60\t22\tFC\tFF\tFF\tFF\t4B\r\n      1944  0CF103A7   00000004    8        17\t1F\t08\t60\tB1\t1F\t08\t4B\r\n      1944  0CF102A7   00000004    8        30\t75\tE0\t2E\t80\tFF\tFF\tFD\r\n      1943  0C3C4D4A   00000004    8        BE\tFF\tFF\t7F\t18\tFF\tFF\t4B\r\n      1943  0CF101A7   00000004    8        68\t00\t97\tCC\t00\t16\t39\t7B\r\n      1942  18F120F0   00000004    8        2B\t75\t60\tB1\tB0\t01\tFF\tFF\r\n      1963  0CF101A7   00000004    8        68\t00\t97\tCC\t00\t16\t39\t7C\r\n      1962  1FFFFFFF   00000004    8        00\t00\tFF\tFF\tFF\tFF\tFF\tFF\r\n      1952  1FFFFFFF   00000004    8        00\t00\tFF\tFF\tFF\tFF\tFF\tFF\r\n      1947  1FFFFFFF   00000004    8        00\t20\tFF\tFF\tFF\tFF\tFF\tFF\r\n      1946  18F121F0   00000004    8     
